vi "angle+count.vi"() -> ()   [LabVIEW 2014]
uses:
  <vilib>/Platform/TimedLoop/XDataNode/timing_clust.ctl
  <vilib>/Platform/TimedLoop/XDataNode/nitl_modes.ctl
  <vilib>/Platform/TimedLoop/XDataNode/wakeup.ctl
  <vilib>/myRIO/Common/Instrument Driver Framework/myRIO v1.0/Encoder/typedefs/Encoder Signal Mode.ctl
  <vilib>/myRIO/Instrument Drivers/Onboard IO/Encoder/typedefs/Encoder Reference.ctl
  <vilib>/myRIO/Common/Instrument Driver Framework/Utilities/typedefs/myRIO Generic Hardware Reference.ctl
  <vilib>/myRIO/Common/Instrument Driver Framework/Utilities/typedefs/Hardware Version Enum.ctl
  <vilib>/myRIO/Common/Instrument Driver Framework/Utilities/typedefs/myRIO v1.0 Reference.ctl
  <vilib>/myRIO/Common/Instrument Driver Framework/Utilities/typedefs/Generic FPGA Reference.ctl
  <vilib>/myRIO/Common/Instrument Driver Framework/myRIO v1.0/Encoder/typedefs/Encoder Channels Enum.ctl
  <vilib>/myRIO/Common/Instrument Driver Framework/myRIO v1.0/Encoder/typedefs/Encoder Configuration v1.0.ctl
  <vilib>/userdefined/High Color/nirio_resource_hc.ctl
  <vilib>/myRIO/Instrument Drivers/Onboard IO/PWM/typedefs/PWM Reference.ctl
  <vilib>/myRIO/Common/Instrument Driver Framework/myRIO v1.0/PWM/typedefs/PWM Channels Enum.ctl
  <vilib>/myRIO/Instrument Drivers/Onboard IO/PWM/typedefs/PWM Configuration.ctl
  <vilib>/myRIO/Common/Instrument Driver Framework/Utilities/vis/Is FPGA Ref Available.vi
  <vilib>/myRIO/Common/Instrument Driver Framework/myRIO v1.0/Encoder/vis/myRIO v1.1 Open Encoder.vi
  <vilib>/myRIO/Instrument Drivers/Onboard IO/Encoder/vis/Read.vi
  <vilib>/myRIO/Common/Instrument Driver Framework/myRIO v1.0/PWM/vis/myRIO v1.1 Open PWM.vi
  <vilib>/myRIO/Instrument Drivers/Onboard IO/PWM/vis/Set Duty Cycle and Frequency.vi
  <vilib>/myRIO/Instrument Drivers/Onboard IO/AI/vis/Read.vi
  <vilib>/myRIO/Common/Instrument Driver Framework/Utilities/vis/Validate Channels.vi
  <vilib>/myRIO/Common/Instrument Driver Framework/myRIO v1.0/Encoder/vis/myRIO v1.0 Reserve Encoder.vi
  <vilib>/myRIO/Instrument Drivers/Onboard IO/DIO/vis/Write.vi
  <vilib>/myRIO/Common/Instrument Driver Framework/myRIO v1.0/PWM/vis/myRIO v1.0 Reserve PWM.vi
  <vilib>/myRIO/Common/Instrument Driver Framework/myRIO v1.0/Encoder/vis/myRIO v1.0 Build MUX Configuration Encoder.vi
  <vilib>/myRIO/Common/Instrument Driver Framework/myRIO v1.0/Resource Manager/vis/myRIO v1.0 Reserve Channel List.vi
  <vilib>/myRIO/Common/Instrument Driver Framework/myRIO v1.0/PWM/vis/myRIO v1.0 Build MUX Configuration PWM.vi
  <vilib>/myRIO/Common/Instrument Driver Framework/myRIO v1.0/Resource Manager/vis/myRIO v1.0 Create Configuration List.vi
  <vilib>/myRIO/Common/Instrument Driver Framework/myRIO v1.0/Resource Manager/vis/myRIO v1.0 Reserve Channel.vi
  <vilib>/myRIO/Common/Instrument Driver Framework/myRIO v1.0/Resource Manager/vis/myRIO v1.0 Unreserve Channel.vi
  <vilib>/myRIO/Common/Instrument Driver Framework/myRIO v1.0/Resource Manager/vis/myRIO v1.0 Build Mutex Name.vi
  <vilib>/myRIO/Instrument Drivers/Onboard IO/AI/vis/Smart Open.vi
  <vilib>/Utility/error.llb/Error Cluster From Error Code.vi
  <vilib>/myRIO/Common/Instrument Driver Framework/myRIO v1.0/AI/vis/myRIO v1.0 Read AI.vi
  <vilib>/Utility/VariantDataType/GetNumericInfo.vi
  <vilib>/myRIO/Common/Instrument Driver Framework/myRIO v1.0/myRIO v1.1 Open.vi
  <vilib>/myRIO/Common/Instrument Driver Framework/Utilities/vis/IO Manager.vi
  <vilib>/myRIO/Common/Instrument Driver Framework/Utilities/vis/Configuration Manager.vi
  <vilib>/myRIO/Common/Instrument Driver Framework/myRIO v1.0/Resource Manager/vis/myRIO v1.0 Configure IO.vi
  <vilib>/myRIO/Common/Instrument Driver Framework/myRIO v1.0/myRIO v1.0 Close.vi
  <vilib>/myRIO/Common/Instrument Driver Framework/myRIO v1.0/Encoder/vis/myRIO v1.0 Configure Encoder.vi
  <vilib>/myRIO/Common/Instrument Driver Framework/myRIO v1.0/Encoder/vis/myRIO v1.0 Read Encoder.vi
  <vilib>/addons/control/pid/pid.llb/PID (DBL).vi
  <vilib>/myRIO/Instrument Drivers/Onboard IO/PWM/vis/Smart Open.vi
  <vilib>/myRIO/Common/Instrument Driver Framework/myRIO v1.0/PWM/vis/myRIO v1.0 Write PWM.vi
  <vilib>/myRIO/Instrument Drivers/Onboard IO/DIO/vis/Smart Open.vi
  <vilib>/myRIO/Common/Instrument Driver Framework/myRIO v1.0/DIO/vis/myRIO v1.0 Write DIO.vi
  <vilib>/platform/TimedLoop/XDataNode/XDataNode.xnode
  <vilib>/myRIO/Express VI/Onboard IO/Encoder/Encoder Express VI.xnode
  <vilib>/myRIO/Instrument Drivers/Onboard IO/Encoder/vis/myRIO Encoder Open.xnode
  <vilib>/myRIO/Express VI/Onboard IO/PWM/PWM Express VI.xnode
  <vilib>/myRIO/Instrument Drivers/Onboard IO/PWM/vis/myRIO PWM Open.xnode
  <vilib>/Platform/TimedLoop/XDataNode/XDNodeRunTimeDep.lvlib
  <vilib>/myRIO/Instrument Drivers/Onboard IO/PWM/PWM.lvlib
  <vilib>/addons/control/pid/NI_PID_pid.lvlib
  <vilib>/myRIO/Instrument Drivers/Onboard IO/Encoder/Encoder.lvlib
  <vilib>/ptbypt/NI_PtbyPt.lvlib
panel:
  in  "行走速度":dbl(slide) scale=-0.01..0.01
  in  "Rorate":dbl
  in  "output range":cluster{"output high":dbl, "output low":dbl}={"output high"=100.0, "output low"=-100.0} {"output low" format="%.3f"; "output high" format="%.3f"}
  out "input":dbl(graph)
  in  "前进后退":dbl(slide) scale=-2.0..2.0
  in  "关闭程序":bool
  in  "电机开关":bool
  out "position_A":i32
  in  "码盘清零":bool
  out "velocity_A":dbl(graph)
  out "position_B":i32
  in  "Reset_B":bool
  out "velocity_B":dbl(graph)
  out "Angluar Rate 2":dbl(graph)
  out "Angluar Rate_average  2":dbl(graph)
  out "Angle_average":dbl(graph)
  out "Angle_org":dbl(graph)
  out "Angluar Rate":dbl
  out "Angluar Rate_average":dbl
  in  "清零":bool
  out "V_In":dbl
  out "output":dbl(graph)
  in  "angle":T1={"proportional gain (Kc)"=1.0, "integral time (Ti, min)"=0.01, "derivative time (Td, min)"=0.0} {"derivative time (Td, min)" format="%.5f"; "integral time (Ti, min)" format="%.5f"; "proportional gain (Kc)" format="%.3f"}
  in  "gyro_bias":dbl
  in  "输出":bool
  in  "position":T1={"proportional gain (Kc)"=1.0, "integral time (Ti, min)"=0.01, "derivative time (Td, min)"=0.0} {"derivative time (Td, min)" format="%.6f"; "integral time (Ti, min)" format="%.5f"; "proportional gain (Kc)" format="%.4f"}
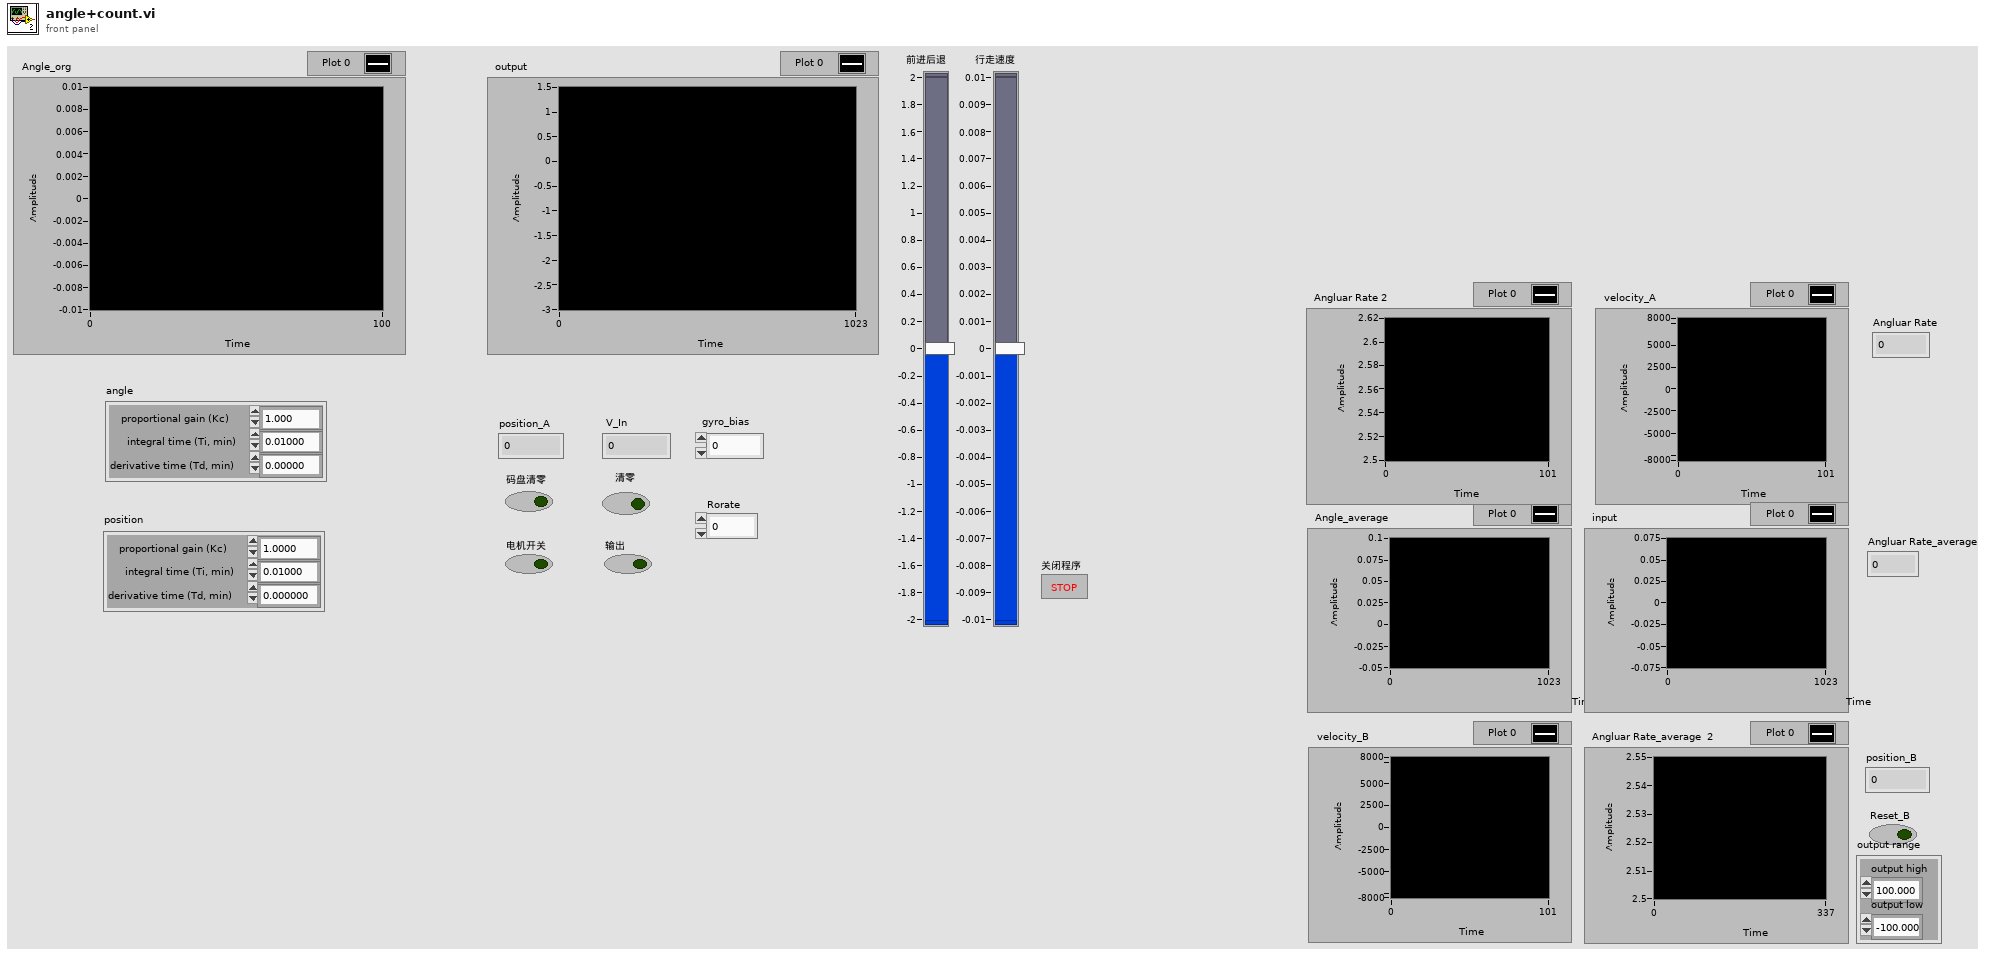
[diagram p1: front panel]
types:
  T1 = cluster{"proportional gain (Kc)":dbl, "integral time (Ti, min)":dbl, "derivative time (Td, min)":dbl}
  T2 = typedef "XDNodeRunTimeDep.lvlib/timing_clust.ctl" = cluster{"Expected End [f-1]":u64, "Actual End [f-1]":u64, "Finished Late? [f-1]":bool, "Expected End [i-1]":u64, "Actual End [i-1]":u64, "Finished Late? [i-1]":bool, "Expected Start [i]":u64, "Actual Start [i]":u64, "Expected Start [f]":u64, "Actual Start [f]":u64, "Source Name":string, "Structure Name":string, "Period":i64, "Deadline":i64, "Offset":i64, "Start":i64, "Priority":i32, "Timeout":i32, "Mode":T3, "Wakeup Reason":T4, "Error":errorcluster, "Source Type":string, "Secondary Source Type":string, "Global End Time":u64, "Global Start Time":u64, "Frame Duration":u64, "Iteration Duration":u64, "Assigned CPU":i32, "I/O Scan Engine Mode":u32}
  T3 = typedef "XDNodeRunTimeDep.lvlib/nitl_modes.ctl" = enum32{"No Change", "Process missed periods, maintain original phase", "Discard missed periods, maintain original phase", "Process missed periods, ignore original phase", "Discard missed periods, ignore original phase"}
  T4 = typedef "XDNodeRunTimeDep.lvlib/wakeup.ctl" = enum32{"Normal", "Aborted", "Asynchronous wakeup", "Timing source error", "Timed loop error", "Timeout"}
  T5 = typedef "Encoder.lvlib/Encoder Reference.ctl" = cluster{"myRIO Reference":T6, "Encoder Channels Enum":T10}
  T6 = typedef "myRIO Generic Hardware Reference.ctl" = cluster{"myRIO Model":T7, "myRIO Hardware Reference":T8}
  T7 = typedef "Hardware Version Enum.ctl" = enum16{"Unknown", "myRIO-1900", "myRIO-1950"}
  T8 = typedef "myRIO v1.0 Reference.ctl" = cluster{"Generic FPGA Reference":T9, "Allow multiple opens":bool}
  T9 = typedef "Generic FPGA Reference.ctl" = refnum<k20>
  T10 = typedef "Encoder Channels Enum.ctl" = enum16{"Not Connected", "C/ENC0", "C/ENC1", "A/ENC", "B/ENC"}
  T11 = typedef "Encoder Signal Mode.ctl" = enum16{"Quadrature phase signal", "Step and direction signal"}
  T12 = typedef "nirio_resource_hc.ctl" = tag
  T13 = typedef "PWM.lvlib/PWM Reference.ctl" = cluster{"myRIO Reference":T6, "PWM Channels Enum":T14, "PWM Configuration":T15}
  T14 = typedef "PWM Channels Enum.ctl" = enum16{"Not Connected", "C/PWM0", "C/PWM1", "A/PWM0", "A/PWM1", "A/PWM2", "B/PWM0", "B/PWM1", "B/PWM2"}
  T15 = typedef "PWM.lvlib/PWM Configuration.ctl" = cluster{"Frequency":dbl, "Duty Cycle":dbl}
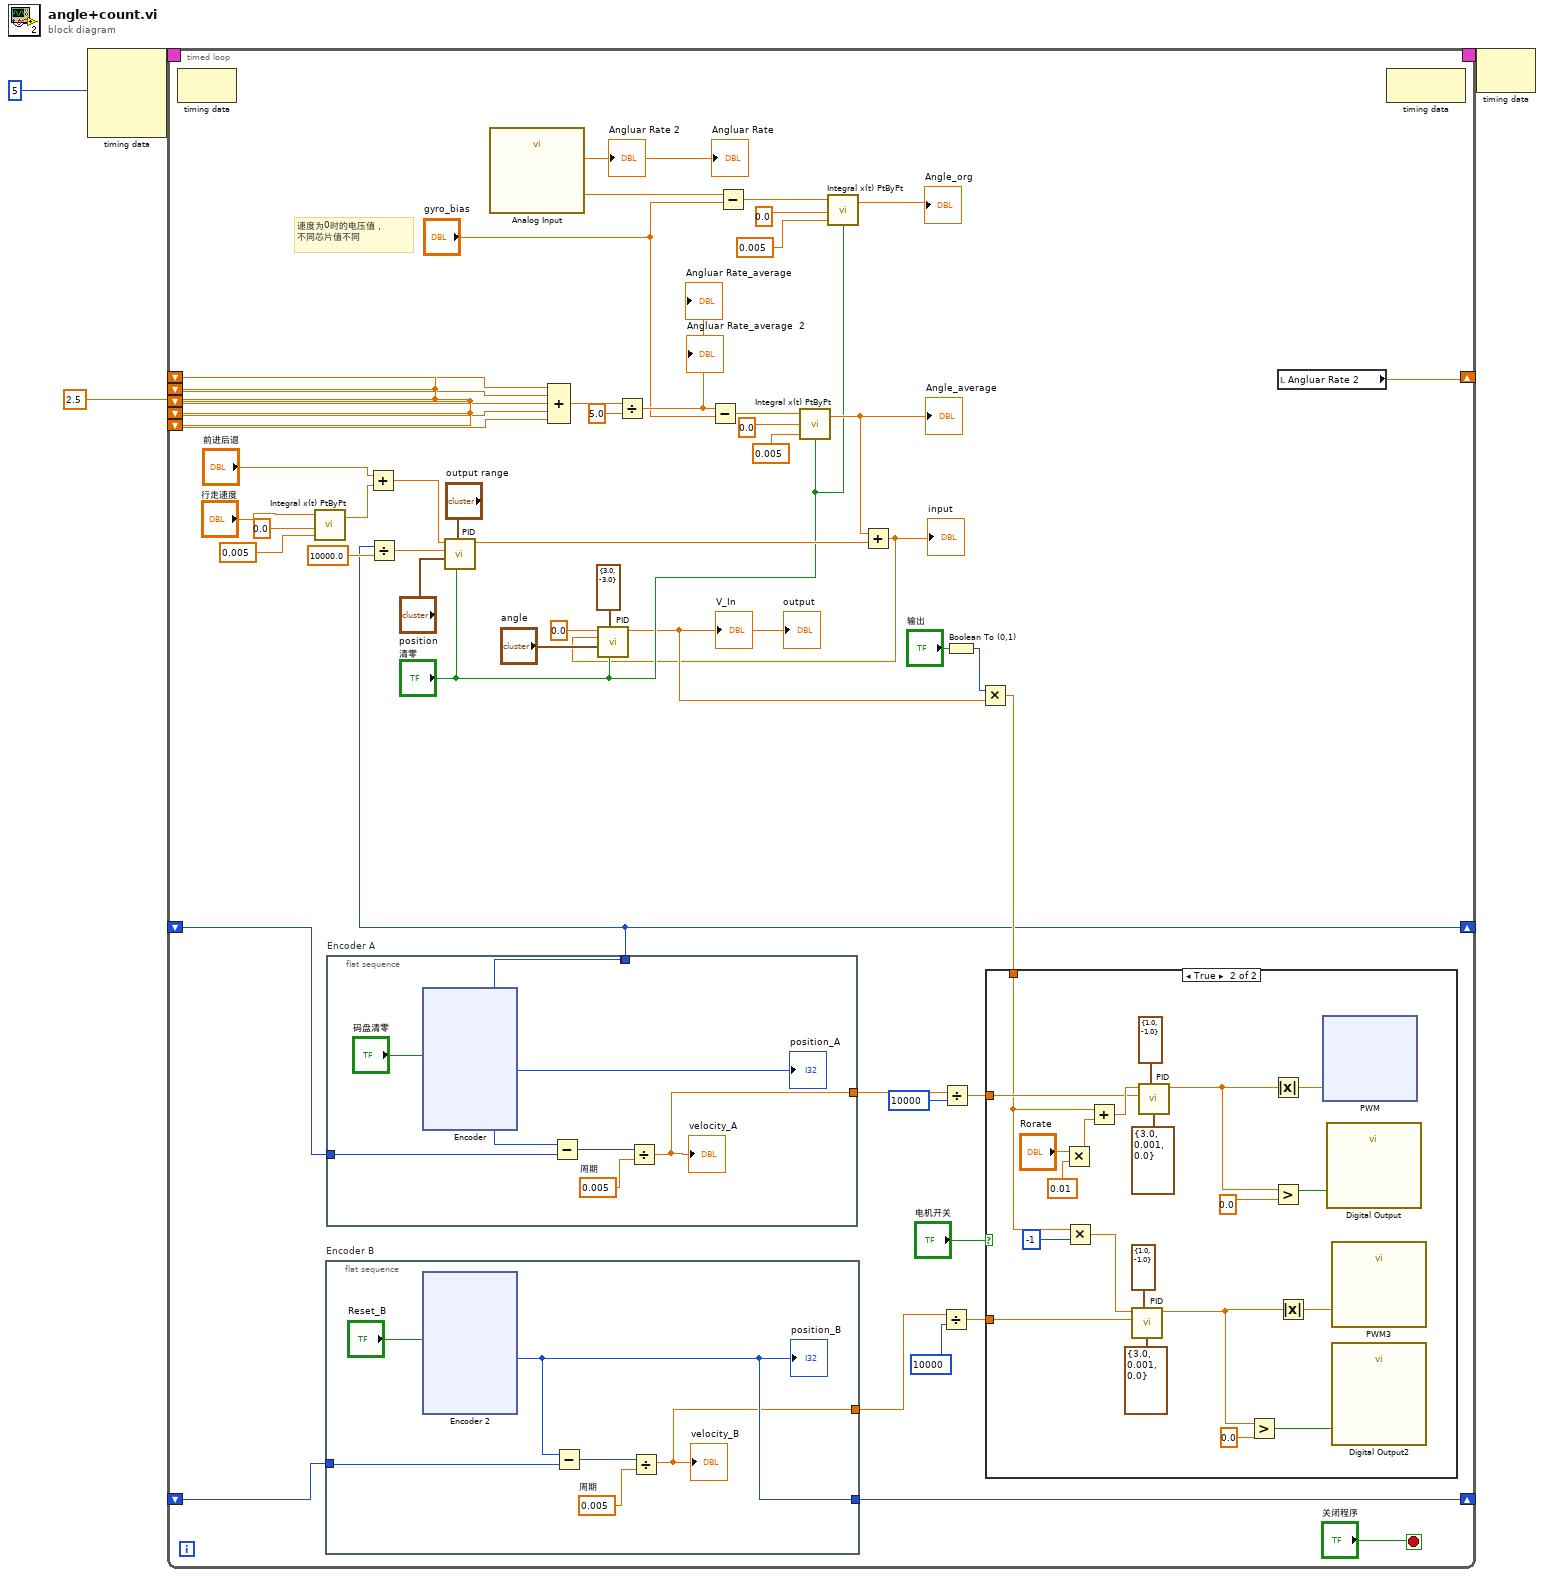
[diagram p0: block diagram]
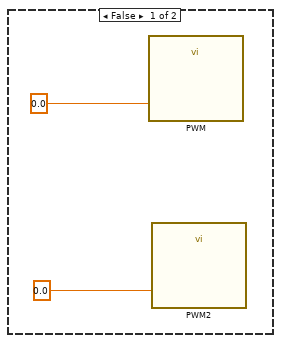
[diagram p2: hidden frame]
diagram:
  w2 = 2.5
  n1 = node-c288(i64 5 ("Period")) -> (w4:T2)  [unwired: 3 in]
  n2 = timed-loop {
    timing: w4 -> [_]
    timing-out: [_] -> w3
    shift-right: [w15] -> _
    shift-left: _ -> [w53]
    shift-right: [w51] -> _
    shift-left: _ -> [w52]
    shift-right: [w41] -> _
    shift-left: w2 -> [w40]
    shift-left: w2 -> [w39]
    shift-left: w2 -> [w38]
    shift-left: w2 -> [w37]
    shift-left: w2 -> [w36]
    stop <- "关闭程序" stop-if-true
    # "速度为0时的电压值，\n不同芯片值不同"
    n3 = node-c288() -> ()  [unwired: 1 in, 1 out]
    n4 = call <vilib>:"Integral x(t) PtByPt.vi"("dt"=0.005, "initial condition"=0.0, "x"="行走速度") -> ("integral x(t)"=w5:dbl)  [unwired: 1 in, 1 out]
    n5 = flat-sequence "Encoder B" {
      tunnel: [w57] -> w51
      tunnel: w52 -> [w60]
      tunnel: [w56] -> w14
      frame #0 {
        w58 = 0.005  # 周期
        n6 = xnode "Encoder 2"("Reset Counter"="Reset_B") -> ("Counter Value"=w57:i32)  [unwired: 1 in, 3 out]
        "position_B" <- w57
        n7 = Subtract(x=w57, y=w60) -> (x-y=w59:i32)
        n8 = Divide(x=w59, y=w58) -> (x/y=w56:dbl)
        "velocity_B" <- w56
      }
    }
    n9 = flat-sequence "Encoder A" {
      tunnel: [w109] -> _
      tunnel: w53 -> [w112]
      tunnel: [w109] -> w15
      tunnel: [w108] -> w23
      frame #0 {
        w110 = 0.005  # 周期
        n10 = xnode "Encoder"("Reset Counter"="码盘清零") -> ("Counter Value"=w109:i32)  [unwired: 1 in, 3 out]
        "position_A" <- w109
        n11 = Subtract(x=w109, y=w112) -> (x-y=w111:i32)
        n12 = Divide(x=w111, y=w110) -> (x/y=w108:dbl)
        "velocity_A" <- w108
      }
    }
    n13 = Add(x="前进后退", y=w5) -> (x+y=w10:dbl)
    n14 = Divide(x=w15, y=10000.0) -> (x/y=w29:dbl)
    n15 = call-poly <vilib>:"PID.vi"("reinitialize? (F)"="清零", "output range"="output range", "PID gains"="position", "process variable"=w29, "setpoint"=w10) -> ("output"=w27:dbl)  [unwired: 5 in, 1 out]
    n16 = call "Analog Input"() -> ("B/AI0 (Pin 3)"=w19:dbl)  [unwired: 26 in, 1 out]
    "Angluar Rate 2" <- w19
    "Angluar Rate" <- w19
    n17 = Compound Arithmetic op=ADD(w40, w39, w38, w37, w36) -> (w50:dbl)
    n18 = Divide(x=w50, y=5.0) -> (x/y=w35:dbl)
    "Angluar Rate_average  2" <- w35
    "Angluar Rate_average" <- w35
    n19 = Subtract(x=w35, y="gyro_bias") -> (x-y=w48:dbl)
    n20 = Subtract(x=w19, y="gyro_bias") -> (x-y=w45:dbl)
    n21 = call <vilib>:"Integral x(t) PtByPt.vi"("initialize"="清零", "dt"=0.005, "initial condition"=0.0, "x"=w48) -> ("integral x(t)"=w26:dbl)  [unwired: 1 out]
    "Angle_average" <- w26
    n22 = call <vilib>:"Integral x(t) PtByPt.vi"("initialize"="清零", "dt"=0.005, "initial condition"=0.0, "x"=w45) -> ("integral x(t)"=→"Angle_org":dbl)  [unwired: 1 out]
    n23 = Add(x=w26, y=w27) -> (x+y=w11:dbl)
    "input" <- w11
    n24 = call-poly <vilib>:"PID.vi"("reinitialize? (F)"="清零", "output range"=cluster{"output high":dbl, "output low":dbl} {"output high"=3.0, "output low"=-3.0}, "PID gains"="angle", "process variable"=w11, "setpoint"=0.0) -> ("output"=w13:dbl)  [unwired: 5 in, 1 out]
    "V_In" <- w13
    "output" <- w13
    n25 = Divide(x=w14, y=10000) -> (x/y=w20:dbl)
    n26 = Divide(x=w23, y=10000) -> (x/y=w21:dbl)
    n27 = Boolean To (0,1)(Boolean="输出") -> (0, 1=w12:i16)
    n28 = Multiply(x=w12, y=w13) -> (x*y=w31:dbl)
    n29 = case shown="True" "电机开关" {
      tunnel: w21 -> [_ w170]
      tunnel: w20 -> [_ w163]
      tunnel: w31 -> [_ w164]
      frame False {
        n30 = call "PWM"("Duty Cycle (0-1)"=0.0) -> ()  [unwired: 26 in, 1 out]
        n31 = call "PWM2"("Duty Cycle (0-1)"=0.0) -> ()  [unwired: 26 in, 1 out]
      }
      frame True {
        n32 = Multiply(x="Rorate", y=0.01) -> (x*y=w165:dbl)
        n33 = Multiply(x=w164, y=-1) -> (x*y=w172:dbl)
        n34 = Add(x=w164, y=w165) -> (x+y=w171:dbl)
        n35 = call-poly <vilib>:"PID.vi"("output range"=cluster{"output high":dbl, "output low":dbl} {"output high"=1.0, "output low"=-1.0}, "PID gains"=T1 {"proportional gain (Kc)"=3.0, "integral time (Ti, min)"=0.001, "derivative time (Td, min)"=0.0}, "process variable"=w163, "setpoint"=w172) -> ("output"=w177:dbl)  [unwired: 6 in, 1 out]
        n36 = call-poly <vilib>:"PID.vi"("output range"=cluster{"output high":dbl, "output low":dbl} {"output high"=1.0, "output low"=-1.0}, "PID gains"=T1 {"proportional gain (Kc)"=3.0, "integral time (Ti, min)"=0.001, "derivative time (Td, min)"=0.0}, "process variable"=w170, "setpoint"=w171) -> ("output"=w178:dbl)  [unwired: 6 in, 1 out]
        n37 = Greater?(x=w177, y=0.0) -> (0:w168:bool)
        n38 = Absolute Value(x=w178) -> (abs(x)=w181:dbl)
        n39 = Greater?(x=w178, y=0.0) -> (0:w176:bool)
        n40 = Absolute Value(x=w177) -> (abs(x)=w179:dbl)
        n41 = xnode "PWM"("Duty Cycle"=w181) -> ()  [unwired: 1 in, 1 out]
        n42 = call "Digital Output"("A/DIO0 (Pin 11)"=w176) -> ()  [unwired: 26 in, 1 out]
        n43 = call "PWM3"("Duty Cycle (0-1)"=w179) -> ()  [unwired: 26 in, 1 out]
        n44 = call "Digital Output2"("B/DIO0 (Pin 11)"=w168) -> ()  [unwired: 26 in, 1 out]
      }
    }
    n45 = local read "Angluar Rate 2"() -> (w41:dbl)
    n46 = node-c288() -> ()  [unwired: 1 in, 1 out]
  }
  n47 = node-c288(w3) -> ()  [unwired: 1 out]
